vi "Waveforms.Start.vi"(8 "error in (no error)":errorcluster, 11 "Cluster in":T1) -> (0 "error out":errorcluster, 3 "Cluster out":T1)   [LabVIEW 2015]
uses:
  Types/Main.StateVariables.ctl
  <vilib>/Utility/miscctls.llb/LVPositionTypeDef.ctl
  Types/Execute.UserEventRefs.ctl
  <vilib>/NI Veristand/Execution/Workspace/SystemStateRegEventRef.ctl
  <vilib>/NI Veristand/Execution/Workspace/Target State Info.ctl
  <vilib>/NI Veristand/Execution/Workspace/Target State.ctl
  <vilib>/NI Veristand/Execution/WaveformStreaming/Waveform Data Watcher Event Data (DBL).ctl
  <vilib>/NI Veristand/Execution/WaveformStreaming/WaveformStreamSpecification.ctl
  NationalInstruments.VeriStand.ClientAPI
  <vilib>/NI Veristand/Execution/Workspace/SystemStateEventRef.ctl
  <vilib>/NI Veristand/Execution/Workspace/WorkspaceAPI.ctl
  Types/UI.Object.ctl
  Types/Waveforms.Info.ctl
  <vilib>/NI Veristand/Execution/WaveformStreaming/Registered Waveform Streams Data Event Refnum (DBL).ctl
  <vilib>/NI Veristand/Execution/WaveformStreaming/WaveformDataWatcherDBL.ctl
  <vilib>/NI Veristand/Execution/WaveformStreaming/WaveformStreamingAPI.ctl
  NationalInstruments.VeriStand
  <vilib>/NI Veristand/Execution/Workspace/NI_VS Workspace ExecutionAPI.lvlib
  <vilib>/NI Veristand/Execution/WaveformStreaming/NI_VS Waveform Streaming Interface.lvlib
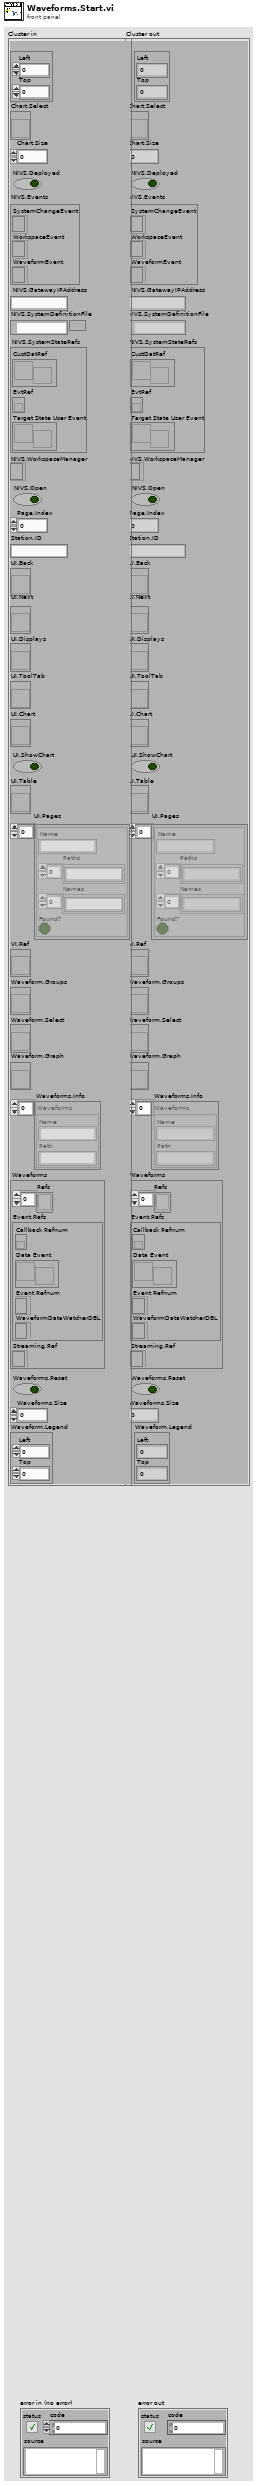
[diagram p1: front panel]
types:
  T1 = typedef "Main.StateVariables.ctl" = cluster{"Chart.Legend":T2, "Chart.Select":refnum<vi>, "Chart.Size":i32, "NIVS.Deployed":bool, "NIVS.Events":T3, "NIVS.GatewayIPAddress":string, "NIVS.SystemDefinitionFile":path, "NIVS.SystemStateRefs":T5, "NIVS.WorkspaceManager":T6, "NIVS.Open":bool, "Page.Index":u32, "Station.ID":string, "UI.Back":refnum<vi>, "UI.Next":refnum<vi>, "UI.Displays":refnum<vi>, "UI.ToolTab":refnum<vi>, "UI.Chart":refnum<vi>, "UI.ShowChart":bool, "UI.Table":refnum<vi>, "UI.Pages":T7[], "VI.Ref":refnum<vi>, "Waveform.Groups":refnum<vi>, "Waveform.Select":refnum<vi>, "Waveform.Graph":refnum<vi>, "Waveforms.Info":T8[], "Waveforms":cluster{"Refs":T9[], "Event.Refs":T10, "Streaming.Ref":T12}, "Waveforms.Reset":bool, "Waveforms.Size":i32, "Waveform.Legend":T2}
  T2 = typedef "LVPositionTypeDef.ctl" = cluster{"Left":i32, "Top":i32}
  T3 = typedef "Execute.UserEventRefs.ctl" = cluster{"SystemChangeEvent":T4, "WorkspaceEvent":refnum<event-registration>, "WaveformEvent":refnum<event-registration>}
  T4 = typedef "NI_VS Workspace ExecutionAPI.lvlib/SystemStateRegEventRef.ctl" = refnum<event-registration>
  T5 = typedef "NI_VS Workspace ExecutionAPI.lvlib/SystemStateEventRef.ctl" = cluster{"CustDatRef":refnum<user-event>, "EvtRef":refnum<k27>, "Target State User Event":refnum<user-event>}
  T6 = typedef "NI_VS Workspace ExecutionAPI.lvlib/WorkspaceAPI.ctl" = refnum<k24>
  T7 = typedef "UI.Object.ctl" = cluster{"Name":string, "Paths":string[], "Names":string[], "Found?":bool}
  T8 = typedef "Waveforms.Info.ctl" = cluster{"Name":string, "Path":string}
  T9 = typedef "NI_VS Waveform Streaming Interface.lvlib/WaveformStreamSpecification.ctl" = refnum<k24>
  T10 = typedef "NI_VS Waveform Streaming Interface.lvlib/Registered Waveform Streams Data Event Refnum (DBL).ctl" = cluster{"Callback Refnum":refnum<k27>, "Data Event":refnum<user-event>, "Event Refnum":refnum<event-registration>, "WaveformDataWatcherDBL":T11}
  T11 = typedef "NI_VS Waveform Streaming Interface.lvlib/WaveformDataWatcherDBL.ctl" = refnum<k24>
  T12 = typedef "NI_VS Waveform Streaming Interface.lvlib/WaveformStreamingAPI.ctl" = refnum<k24>
  T13 = cluster{"Waveform.Refs":T9[], "WaveformStreaming.Event.Refs":T10, "WaveformStreaming.Ref":T12}
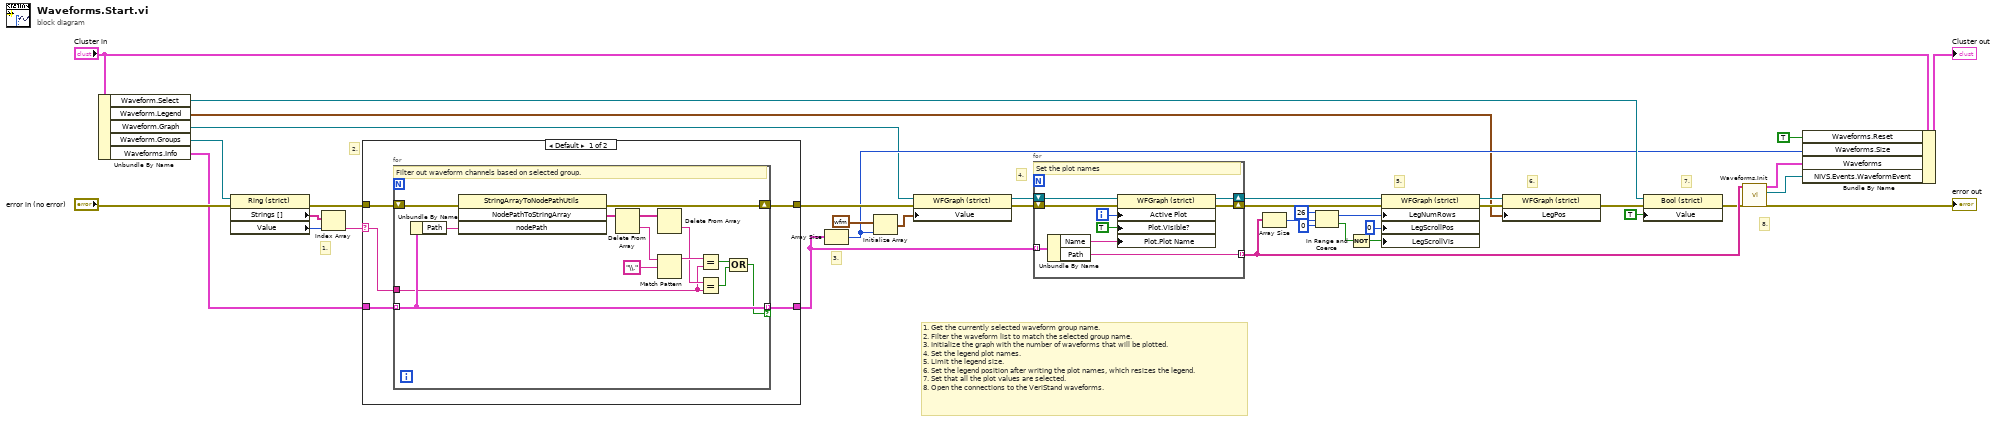
[diagram p0: block diagram]
diagram:
  # "4."
  # "3."
  # "1. Get the currently selected waveform group name.\n2. Filter the waveform list to match the selected group name.\n3. Initialize the graph with the number of waveforms that will be plotted.\n4. Set the legend plot names.\n5. Limit the legend size.\n6. Set the legend position after writing the plot names, which resizes the legend.\n7. Set that all the plot values are selected.\n8. Open the connections to the VeriStand waveforms."
  # "8."
  # "7."
  # "6."
  # "5."
  # "2."
  # "1."
  n1 = Unbundle By Name("Cluster in") -> ("Waveform.Select"=w8:refnum<vi>, "Waveform.Legend"=w2:T2, "Waveform.Graph"=w1:refnum<vi>, "Waveform.Groups"=w35:refnum<vi>, "Waveforms.Info"=w22:T8[])
  n2 = property class="Ring (strict)"(reference=w35, error in="error in (no error)") -> (error out=w20:errorcluster, "Strings []"=w37:string[], "Value"=w38:u8)  [unwired: 1 out]
  n3 = Index Array(array=w37, index=w38) -> (element=w29:string)
  n4 = case shown="Default" w29 {
    selector: w29 -> [w40 _]
    tunnel: w22 -> [w43 w59]
    tunnel: [w39 w59] -> w16
    tunnel: w20 -> [w42 w58]
    tunnel: [w41 w58] -> w18
    frame Default {
      n5 = for {
        tunnel: w43 -> [w52] mode=indexing
        shift-right: [w53] -> w41
        shift-left: w42 -> [w56]
        tunnel: w40 -> [w44]
        tunnel: [w52] -> w39 mode=indexing if=w45
        # "Filter out waveform channels based on selected group."
        n6 = Unbundle By Name(w52) -> ("Path"=w57:string)
        n7 = invoke class="StringArrayToNodePathUtils" method="NodePathToStringArray"(error in=w56, "nodePath"=w57) -> (error out=w53:errorcluster, "NodePathToStringArray"=w55:string[])  [unwired: 2 in, 2 out]
        n8 = Delete From Array(array=w55) -> (deleted portion=w51:string, array with subset deleted=w54:string[])  [unwired: 2 in]
        n9 = Delete From Array(array=w54) -> (deleted portion=w48:string)  [unwired: 2 in, 1 out]
        n10 = Match Pattern(string=w51, regular expression="\\.") -> (before substring=w49:string)  [unwired: 1 in, 3 out]
        n11 = Equal?(x=w49, y=w44) -> (x = y?=w47:bool)
        n12 = Equal?(x=w48, y=w44) -> (x = y?=w46:bool)
        n13 = Compound Arithmetic op=OR(w47, w46) -> (w45:bool)
      }
    }
    frame "All" {
    }
  }
  n14 = Array Size(array=w16) -> (size(s)=w6:i32)
  n15 = Initialize Array(waveform(dbl) {"t0"=timestamp(0 s since 1904-01-01), "dt"=1.0, "Y"=[]} ("output waveform"), w6) -> (w14:waveform(dbl)[])
  n16 = property class="WFGraph (strict)"(reference=w1, error in=w18, "Value"=w14) -> (reference out=w17:refnum<vi>, error out=w19:errorcluster)
  n17 = for {
    shift-right: [w66] -> w28
    shift-left: w19 -> [w67]
    tunnel: w16 -> [w64] mode=indexing
    tunnel: [w62] -> w27 mode=indexing
    shift-right: [w61] -> w21
    shift-left: w17 -> [w68]
    i -> [w65]
    # "Set the plot names"
    n18 = Unbundle By Name(w64) -> ("Name"=w63:string, "Path"=w62:string)
    n19 = property class="WFGraph (strict)"(reference=w68, error in=w67, "Active Plot"=w65, "Plot.Visible?"=TRUE ("Plot.Visible"), "Plot.Plot Name"=w63) -> (reference out=w61:refnum<vi>, error out=w66:errorcluster)
  }
  n20 = Array Size(array=w27) -> (size(s)=w26:i32)
  n21 = In Range and Coerce(upper limit=26, x=w26, lower limit=0) -> (coerced(x)=w23:i32, In Range?=w12:bool)
  n22 = Not(x=w12) -> (.not. x?=w11:bool)
  n23 = property class="WFGraph (strict)"(reference=w21, error in=w28, "LegNumRows"=w23, "LegScrollPos"=u32 0 ("Legend:Scroll Position"), "LegScrollVis"=w11) -> (reference out=w5:refnum<vi>, error out=w4:errorcluster)
  n24 = property class="WFGraph (strict)"(reference=w5, error in=w4, "LegPos"=w2) -> (error out=w3:errorcluster)  [unwired: 1 out]
  n25 = property class="Bool (strict)"(reference=w8, error in=w3, "Value"=TRUE) -> (error out=w9:errorcluster)  [unwired: 1 out]
  n26 = call "Waveforms.Init.vi"("error in"=w9, "Channel.Paths"=w27) -> ("error out"=→"error out":errorcluster, "WaveformStreaming.Event"=w34:refnum<event-registration>, "Waveforms"=w31:T13)  [unwired: 7 in]
  n27 = Bundle By Name(cluster="Cluster in", "Waveforms.Reset"=TRUE, "Waveforms.Size"=w6, "Waveforms"=w31, "NIVS.Events.WaveformEvent"=w34) -> (→"Cluster out":T1)
